vi "CST_AnalysisData.vi"() -> (0 "Analysis Data":T1={"Status (Codes)"=[], "Data (Codes)"=[], "Temp - Data (Volts)"=[], "FFT"={"FFT Data"=[], "Table Col Hdrs"=["SNR (dBFS)", "SNRD(dB)", "THD (dBc)", "SFDR (dBc)", "ENOB", "enob", "# of Harmonics (SNR)", "Worst Spur (dB)", "2nd HD (dBc)", "3rd HD (dBc)", "4th HD (dBc)", "5th HD (dBc)", "Fundamental (dB)", "", "PGA Setting", "CMRR"], "Table Row Hdrs"=[], "Analysis Data"=[], "CMRR/BW Table"=[]}, "Histogram"={"Histogram Data"=[], "Table Col Hdrs"=["SNR (dBFS)", "SNRD(dB)", "THD (dBc)", "SFDR (dBc)", "ENOB", "enob", "# of Harmonics (SNR)", "Worst Spur (dB)", "2nd HD (dBc)", "3rd HD (dBc)", "4th HD (dBc)", "5th HD (dBc)", "Fundamental (dB)", "", "PGA Setting", "CMRR"], "Table Row Hdrs"=[], "Analysis Data"=[]}, "Scope"={"Table Col Hdrs"=[], "Table Row Hdrs"=["SNR (dBFS)", "SNRD(dB)", "THD (dBc)", "SFDR (dBc)", "ENOB", "enob", "# of Harmonics (SNR)", "Worst Spur (dB)", "2nd HD (dBc)", "3rd HD (dBc)", "4th HD (dBc)", "5th HD (dBc)", "Fundamental (dB)", "", "PGA Setting", "CMRR"], "Analysis Data"=[]}, "ECG"={"AUX/LEAD"=[], "Chest Leads"=[], "Graph Labels (current)"=[]}, "Respiration"=[]})   [LabVIEW 2010]
uses:
  Controls/Shift Registers/TYP_AnalysisData.ctl
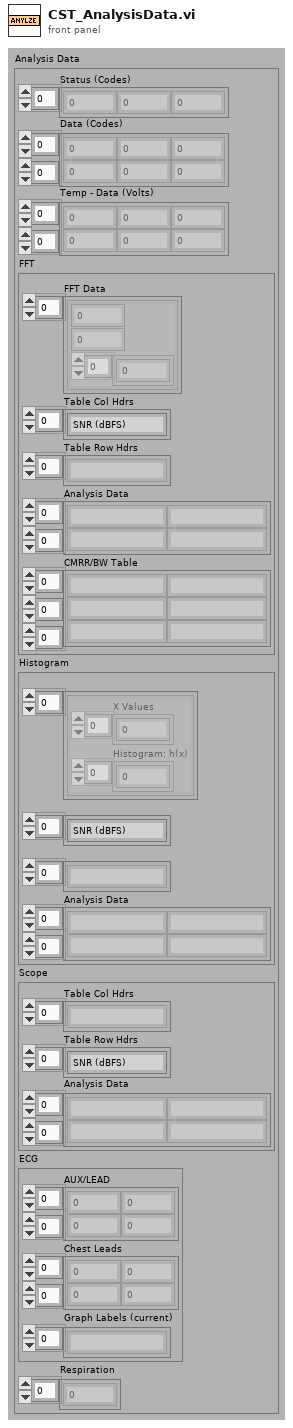
[diagram p1: front panel]
types:
  T1 = typedef "TYP_AnalysisData.ctl" = cluster{"Status (Codes)":i32[], "Data (Codes)":i32[][], "Temp - Data (Volts)":dbl[][], "FFT":cluster{"FFT Data":cluster{i32, dbl, dbl[]}[], "Table Col Hdrs":string[], "Table Row Hdrs":string[], "Analysis Data":string[][], "CMRR/BW Table":string[][][]}, "Histogram":cluster{"Histogram Data":cluster{"X Values":dbl[], "Histogram: h(x)":i32[]}[], "Table Col Hdrs":string[], "Table Row Hdrs":string[], "Analysis Data":string[][]}, "Scope":cluster{"Table Col Hdrs":string[], "Table Row Hdrs":string[], "Analysis Data":string[][]}, "ECG":cluster{"AUX/LEAD":dbl[][], "Chest Leads":dbl[][], "Graph Labels (current)":string[]}, "Respiration":dbl[]}
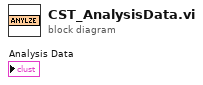
[diagram p0: block diagram]
diagram:
